vi "LV2Global_UsingTemplate.vi"(6 "Variant in":variant, 7 "Shift Pressed?":bool, 8 "error in (no error)":errorcluster, 10 "QD Combo Box Ref":refnum<vi>, 11 "QD Launch VI Ref":refnum<vi>) -> (0 "error out":errorcluster, 4 "Variant out":variant)   [LabVIEW 2014]
doc: "This will create a new LV2 global with a selected constant or control data type. LV2 global will be created using the template file(.vit). Modify the template file to add cases and do other operations.\n\nDefault Shortcut - [3]"
panel:
  in  "Undo Name":string="Quick Drop Keyboard Shortcut"
  # "Do not change the connector pane of this VI.\n\nSee the block diagram for directions on how to use this template."
  # "Specify the name of the Undo transaction"
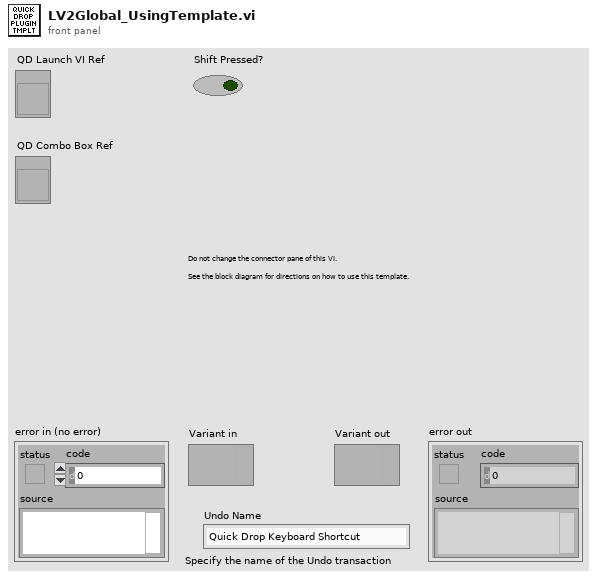
[diagram p1: front panel]
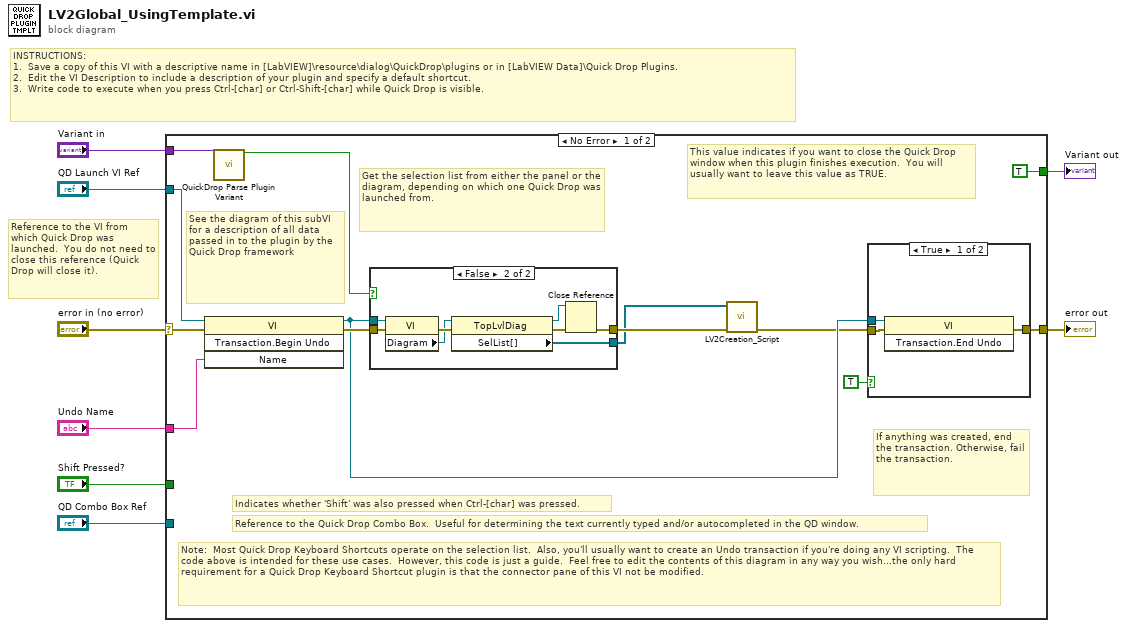
[diagram p0: block diagram]
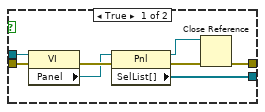
[diagram p2: hidden frame]
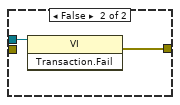
[diagram p3: hidden frame]
diagram:
  # "Reference to the VI from which Quick Drop was launched.  You do not need to close this reference (Quick Drop will close it)."
  # "INSTRUCTIONS:\n1.  Save a copy of this VI with a descriptive name in [LabVIEW]\\resource\\dialog\\QuickDrop\\plugins or in [LabVIEW Data]\\Quick Drop Plugins.\n2.  Edit the VI Description to include a description of your plugin and specify a default shortcut. \n3.  Write code to execute when you press Ctrl-[char] or Ctrl-Shift-[char] while Quick Drop is visible."
  n1 = case shown="No Error" "error in (no error)" {
    selector: "error in (no error)" -> [w21 w43]
    tunnel: [w17 w43] -> w7
    tunnel: "QD Launch VI Ref" -> [w20 _]
    tunnel: "Shift Pressed?" -> [_ _]
    tunnel: "QD Combo Box Ref" -> [_ _]
    tunnel: "Variant in" -> [w13 _]
    tunnel: "Undo Name" -> [w19 _]
    tunnel: [TRUE _] -> w1
    frame No Error {
      # "Note:  Most Quick Drop Keyboard Shortcuts operate on the selection list.  Also, you'll usually want to create an Undo transaction if you're doing any VI scripting.  The code above is intended for these use cases.  However, this code is just a guide.  Feel free to edit the contents of this diagram in any way you wish...the only hard requirement for a Quick Drop Keyboard Shortcut plugin is that the connector pane of this VI not be modified."
      # "Get the selection list from either the panel or the diagram, depending on which one Quick Drop was launched from."
      # "If anything was created, end the transaction. Otherwise, fail the transaction."
      # "This value indicates if you want to close the Quick Drop window when this plugin finishes execution.  You will usually want to leave this value as TRUE."
      # "See the diagram of this subVI for a description of all data passed in to the plugin by the Quick Drop framework"
      # "Reference to the Quick Drop Combo Box.  Useful for determining the text currently typed and/or autocompleted in the QD window."
      # "Indicates whether 'Shift' was also pressed when Ctrl-[char] was pressed."
      n2 = invoke class="VI" method="Transaction.Begin Undo"(reference=w20, error in=w21, "Name"=w19) -> (reference out=w14:refnum<vi>, error out=w15:errorcluster)  [unwired: 1 in, 2 out]
      n3 = call <vilib>:"QuickDrop Parse Plugin Variant.vi"("QDKS Variant in"=w13) -> ("QD Launch VI Panel?"=w12:bool)  [unwired: 12 in, 2 out]
      n4 = case shown="False" w12 {
        tunnel: w15 -> [w29 w37]
        tunnel: w14 -> [w28 w36]
        tunnel: [w23 w31] -> w11
        tunnel: [w22 w30] -> w9
        frame True {
          n5 = property class="VI"(reference=w28, error in=w29) -> (error out=w27:errorcluster, "Panel"=w26:refnum<vi>)  [unwired: 1 out]
          n6 = property class="Pnl"(reference=w26, error in=w27) -> (reference out=w24:refnum<vi>, error out=w25:errorcluster, "SelList[]"=w22:refnum<vi>[])
          n7 = Close Reference(reference=w24, error in (no error)=w25) -> (error out=w23:errorcluster)
        }
        frame False {
          n8 = property class="VI"(reference=w36, error in=w37) -> (error out=w35:errorcluster, "Diagram"=w34:refnum<vi>)  [unwired: 1 out]
          n9 = property class="TopLvlDiag"(reference=w34, error in=w35) -> (reference out=w32:refnum<vi>, error out=w33:errorcluster, "SelList[]"=w30:refnum<vi>[])
          n10 = Close Reference(reference=w32, error in (no error)=w33) -> (error out=w31:errorcluster)
        }
      }
      n11 = call "LV2Creation_Script.vi"("error in (no error)"=w11, "SelList[]"=w9) -> ("error out"=w10:errorcluster)  [unwired: 9 in]
      n12 = case shown="True" TRUE {
        tunnel: w14 -> [w39 w41]
        tunnel: [w40 w42] -> w17
        tunnel: w10 -> [w38 _]
        frame True {
          n13 = invoke class="VI" method="Transaction.End Undo"(reference=w39, error in=w38) -> (error out=w40:errorcluster)  [unwired: 1 in, 2 out]
        }
        frame False {
          n14 = invoke class="VI" method="Transaction.Fail"(reference=w41) -> (error out=w42:errorcluster)  [unwired: 2 in, 2 out]
        }
      }
    }
    frame Error {
    }
  }
  "error out" <- w7
  "Variant out" <- w1
